vi "PointNode_Create.vi"(0 "reference":refnum<class "PointNode.lvclass">, 5 "error in (no error)":errorcluster, 6 "GoopReferenceIn":T1) -> (14 "reference out":refnum<class "PointNode.lvclass">, 16 "# of objects":i32, 19 "error out":errorcluster)   [LabVIEW 2014, in "PointNode.lvclass"]
doc: "Creates and initializes a new PointNode object.\n\nThis object should be destroyed using a PointNode destructor VI or a virtual base class destructor VI.\n\n[GOOP 2.1]"
uses:
  <resource>/Framework/Providers/Open_GDS/UML/PointNode_class/PointNode.lvclass
  <resource>/Framework/Providers/Open_GDS/UML/AbstractNode_class/ObjectReference.ctl
  <resource>/Framework/Providers/Open_GDS/UML/General/Point/Point Point2D.ctl
  <resource>/Framework/Providers/Open_GDS/UML/AbstractNode_class/AbstractNode.lvclass
panel:
  # "The input reference should only\nbe wired when this method is called\nby a sub class constructor."
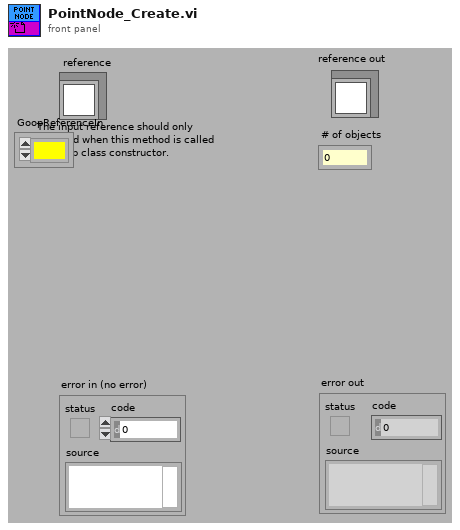
[diagram p1: front panel]
types:
  T1 = typedef "AbstractNode.lvclass/ObjectReference.ctl" = refnum<k1>
  T2 = typedef "Point Point2D.ctl" = cluster{"x":dbl, "y":dbl}
  T3 = typedef "PointNode.lvclass/ObjectAttributes.ctl" = cluster{"Base class":T4, "point":T2}
  T4 = typedef "AbstractNode.lvclass/ObjectAttributes.ctl" = cluster{"parent":refnum<class "AbstractNode.lvclass">, "children":refnum<class "AbstractNode.lvclass">[], "Hidden":bool}
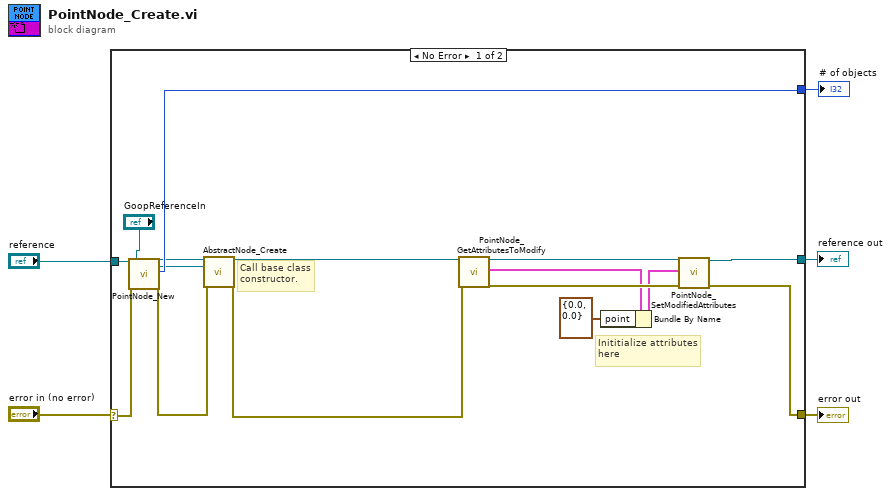
[diagram p0: block diagram]
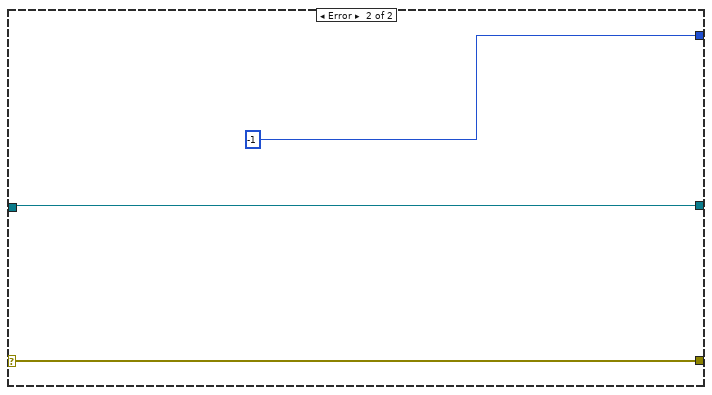
[diagram p2: hidden frame]
diagram:
  n1 = case shown="No Error" "error in (no error)" {
    selector: "error in (no error)" -> [w21 w23]
    tunnel: [w10 w22] -> w5
    tunnel: [w9 w23] -> w4
    tunnel: [w20 -1 ("Nr of open handles")] -> w3
    tunnel: "reference" -> [w19 w22]
    frame No Error {
      # "Inititialize attributes\nhere"
      # "Call base class\nconstructor."
      n2 = call <resource>:"PointNode_New.vi"("reference in"=w19, "error in (no error)"=w21, "GoopReferenceIn"="GoopReferenceIn") -> ("GoopReferenceOut"=w6:T1, "reference out"=w15:refnum<class "PointNode.lvclass">, "# of objects"=w20:i32, "error out"=w18:errorcluster)  [unwired: 2 in, 11 out]
      n3 = call <resource>:"AbstractNode_Create.vi"("reference"=w15, "error in (no error)"=w18, "GoopReferenceIn"=w6) -> ("reference out"=w14:refnum<class "PointNode.lvclass">, "error out"=w16:errorcluster)  [unwired: 15 out]
      n4 = call <resource>:"PointNode_GetAttributesToModify.vi"("reference in"=w14, "error in (no error)"=w16) -> ("reference out"=w13:refnum<class "PointNode.lvclass">, "Attributes"=w12:T3, "error out"=w17:errorcluster)  [unwired: 1 in, 14 out]
      n5 = Bundle By Name(cluster=w12, "point"=T2 {"x"=0.0, "y"=0.0}) -> (w11:T3)
      n6 = call <resource>:"PointNode_SetModifiedAttributes.vi"("reference in"=w13, "Attributes"=w11, "error in (no error)"=w17) -> ("reference out"=w10:refnum<class "PointNode.lvclass">, "error out"=w9:errorcluster)  [unwired: 3 in, 12 out]
    }
    frame Error {
    }
  }
  "error out" <- w4
  "reference out" <- w5
  "# of objects" <- w3
